vi "加标体积写入.vi"(7 "是否启用通讯通知":bool, 8 "error in (no error)":errorcluster, 10 "加标体积":sgl, 11 "Slave ID":T1) -> (0 "error out":errorcluster)   [LabVIEW 2016, in "质控单元V1.lvlib"]
uses:
  <vilib>/Plasmionique/MB Master/MB_Master/MB_Master.lvclass
  <vilib>/Plasmionique/MB Master/MB Master.lvlib
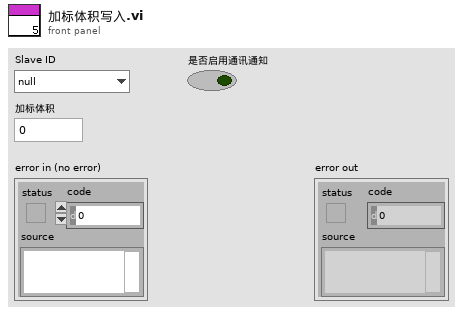
[diagram p1: front panel]
types:
  T1 = typedef "质控单元V1.lvlib/质控slave id.ctl" = enum16{"null", "氨氮", "总磷", "CODMn", "CODCr", "总氮"}
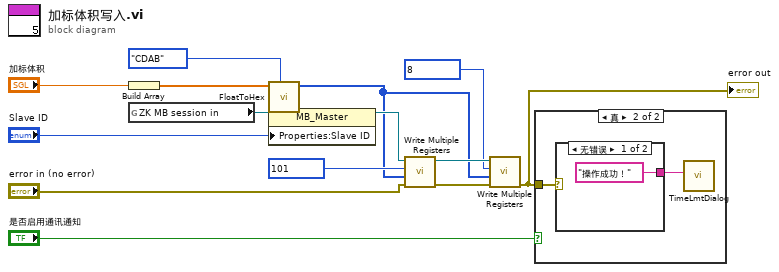
[diagram p0: block diagram]
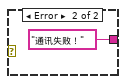
[diagram p3: hidden frame]
diagram:
  n1 = Build Array("加标体积") -> (w9:sgl[])
  n2 = global read "ZK非断电保存全局变量.vi" "ZK MB session in"() -> (w13:refnum<class "MB_Master.lvclass">)
  n3 = call "FloatToHex.vi"("转换类型"=enum16{"DCBA", "CDAB"}."CDAB", "浮点数"=w9) -> ("CDAB整形输出"=w2:u16[])  [unwired: 9 in]
  n4 = property class="MB_Master"(reference=w13, "Properties:Slave ID"="Slave ID") -> (reference out=w11:refnum<class "MB_Master.lvclass">)  [unwired: 1 in, 1 out]
  n5 = call <vilib>:"Write Multiple Registers.vi"("error in (no error)"="error in (no error)", "values"=w2, "starting address"=u16 101, "MB session in"=w11) -> ("error out"=w6:errorcluster, "MB session out"=w4:refnum<class "MB_Master.lvclass">)  [unwired: 6 in]
  n6 = call <vilib>:"Write Multiple Registers.vi"("error in (no error)"=w6, "values"=w2, "starting address"=u16 8, "MB session in"=w4) -> ("error out"=w5:errorcluster)  [unwired: 6 in, 1 out]
  "error out" <- w5
  n7 = case shown="真" "是否启用通讯通知" {
    tunnel: w5 -> [_ w16]
    frame False {
    }
    frame True {
      n8 = case shown="无错误" w16 {
        tunnel: ["操作成功！" "通讯失败！"] -> w15
        frame No Error {
        }
        frame Error {
        }
      }
      n9 = call "TimeLmtDialog.vi"("Infoin"=w15) -> ()  [unwired: 11 in]
    }
  }
